vi "Platform Names.vi"(8 "error in (no error)":errorcluster, 11 "TargetPluginManager in":refnum<class "TargetPluginManager.lvclass">) -> (0 "error out":errorcluster, 2 "Platforms":string[](array[string]), 3 "TargetPluginManager out":refnum<class "TargetPluginManager.lvclass">)   [LabVIEW 2020, in "PicoG-Core.lvlib" / "TargetPluginManager.lvclass"]
uses:
  TargetPluginManager.lvclass
  TargetPluginManager.lvclass/TargetPluginManager.ctl
  DeployTarget/DeployTarget.lvclass
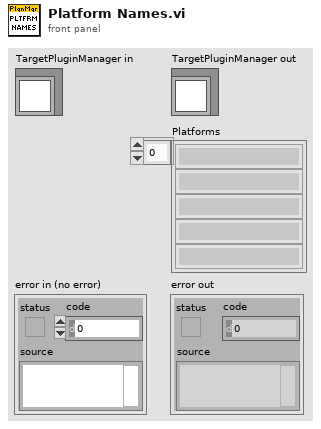
[diagram p1: front panel]
types:
  T1 = typedef "PicoG-Core.lvlib/TargetPluginManager.lvclass/Ref Data.ctl" = cluster{"Targets":refnum<class "DeployTarget.lvclass">[], "Last Target":refnum<class "DeployTarget.lvclass">, "Last Resource":refnum<class "DeployResource.lvclass">}
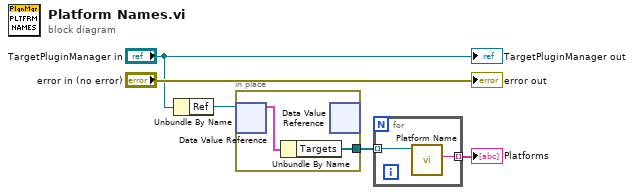
[diagram p0: block diagram]
diagram:
  n1 = Unbundle By Name("TargetPluginManager in") -> ("Ref"=w4:refnum<data-value>)
  n2 = in-place {
    in-place-border: [w6] -> w2
    n3 = in-place-dvr #1(w4) -> (w7:T1)  [unwired: 1 out]
    n4 = Unbundle By Name(w7) -> ("Targets"=w6:refnum<class "DeployTarget.lvclass">[])
    n5 = in-place-dvr #1() -> ()  [unwired: 1 in, 2 out]
  }
  n6 = for {
    tunnel: w2 -> [w9] mode=indexing
    tunnel: [w8] -> w1 mode=indexing
    n7 = call-dynamic "Platform Name.vi"("DeployTarget in"=w9) -> ("Platform Name"=w8:string)  [unwired: 8 in, 2 out]
  }
  "Platforms" <- w1
  "error out" <- "error in (no error)"
  "TargetPluginManager out" <- "TargetPluginManager in"
